vi "Write Single Register.vi"(8 "error in (no error)":errorcluster, 9 "Write Value":u16, 10 "Write address":u16, 11 "Modbus in":refnum<class "Modbus.lvclass">) -> (0 "error out":errorcluster, 3 "Modbus out":refnum<class "Modbus.lvclass">)   [LabVIEW 2023, in "HardwareAbstractionLayer_LVOOP.lvlib" / "Modbus.lvclass"]
uses:
  Modbus.lvclass
  Modbus.lvclass/Modbus.ctl
  <vilib>/NI/Modbus Library/API/Master/Modbus Master.lvclass
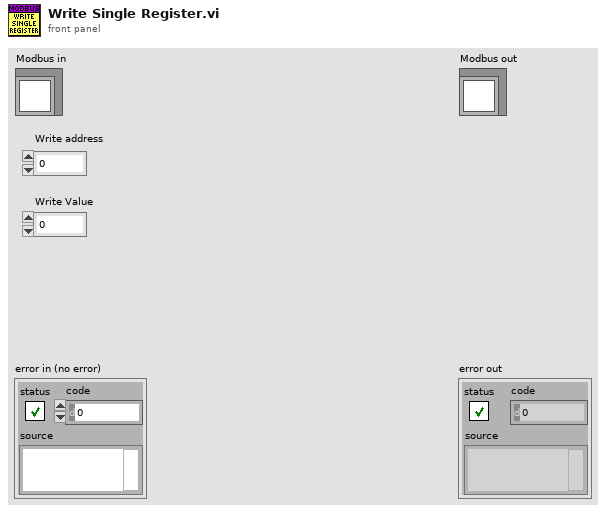
[diagram p1: front panel]
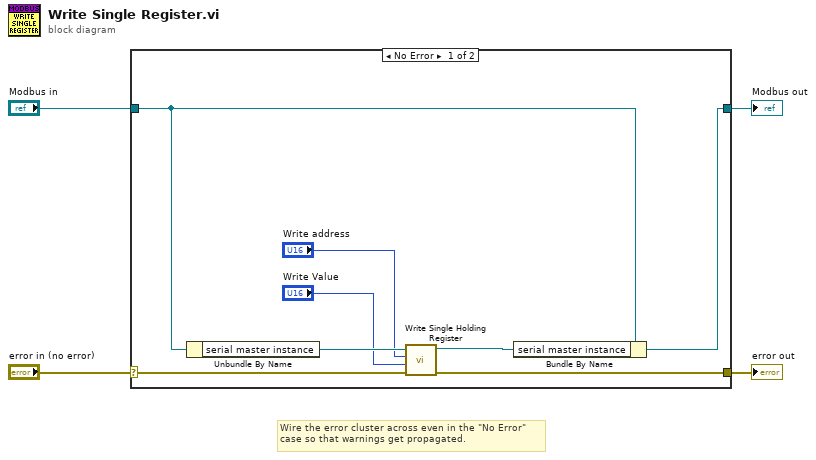
[diagram p0: block diagram]
diagram:
  # "Wire the error cluster across even in the \"No Error\"\ncase so that warnings get propagated."
  n1 = case shown="No Error" "error in (no error)" {
    selector: "error in (no error)" -> [w11 w14]
    tunnel: [w10 w14] -> w3
    tunnel: [w8 w13] -> w1
    tunnel: "Modbus in" -> [w9 w13]
    frame No Error {
      n2 = Unbundle By Name(w9) -> ("serial master instance"=w12:refnum<class "Modbus Master.lvclass">)
      n3 = call-dynamic "Write Single Holding Register.vi"("error in"=w11, "register to write"="Write Value", "address"="Write address", "Modbus master in"=w12) -> ("error out"=w10:errorcluster, "Modbus master out"=w7:refnum<class "Modbus Master.lvclass">)  [unwired: 6 in]
      n4 = Bundle By Name(cluster=w9, "serial master instance"=w7) -> (w8:refnum<class "Modbus.lvclass">)
    }
    frame Error {
    }
  }
  "error out" <- w3
  "Modbus out" <- w1
